vi "EMD8216 counter mask read.vi"(10 "port":u8, 11 "CardID":u32) -> (1 "channel":u8, 3 "error_code":u32)   [LabVIEW 2009, in "EMD8216_64.lvlib"]
doc: "EMD8216Status EMD8216_counter_mask_read(u32 CardID,u8 port,u8 *channel);"
uses:
  EMD8216_64.lvlib
  <userlib>/EMD8216_64/EMD8216_64.dll
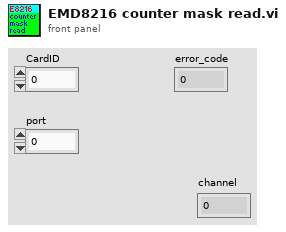
[diagram p1: front panel]
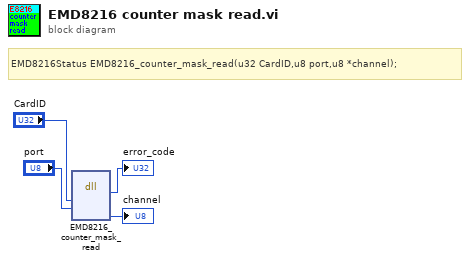
[diagram p0: block diagram]
diagram:
  # "EMD8216Status EMD8216_counter_mask_read(u32 CardID,u8 port,u8 *channel);"
  n1 = dll-call lib="C:/Program Files/National Instruments/LabVIEW 2017/user.lib/EMD8216_64/EMD8216_64.*" fn="EMD8216_counter_mask_read"("CardID"="CardID", "port"="port") -> ("return type"=→"error_code":u32, "channel"=→"channel":u8)  [unwired: 6 in, 2 out]
